vi "Get_LAN_Portnumber.vi"(8 "error in (no error)":errorcluster, 11 ".NET Reference in":refnum<k24>) -> (0 "error out":errorcluster, 1 "portnum":i32, 3 "Reference out":refnum<k24>)   [LabVIEW 2017]
uses:
  C:/Users/Ssantec_Test/Documents/Instrument_DLL_Sample_Labview_20220902_Ver1.2.2/DLL/x86/InstrumentDLL.dll
  DLL/x86/InstrumentDLL.dll
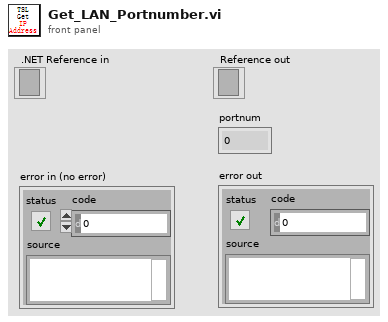
[diagram p1: front panel]
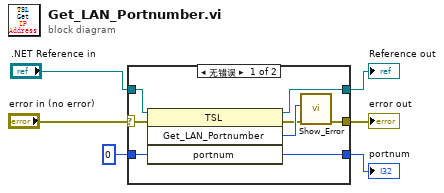
[diagram p0: block diagram]
diagram:
  n1 = case shown="无错误" "error in (no error)" {
    selector: "error in (no error)" -> [w7 w16]
    tunnel: ".NET Reference in" -> [w14 w17]
    tunnel: [w13 w17] -> w5
    tunnel: [w8 w16] -> w4
    tunnel: [w12 w15] -> w3
    tunnel: 0 ("portnum") -> [w11 w15]
    frame No Error {
      n2 = invoke on="调用节点" class="TSL" method="Get_LAN_Portnumber"(reference=w14, error in=w7, "portnum"=w11) -> (reference out=w13:refnum<k24>, error out=w9:errorcluster, "Get_LAN_Portnumber"=w10:i32, "portnum"=w12:i32)  [unwired: 1 in]
      n3 = call "Show_Error.vi"("error in (no error)"=w9, "Error"=w10) -> ("error out"=w8:errorcluster)  [unwired: 9 in]
    }
    frame Error {
    }
  }
  "Reference out" <- w5
  "error out" <- w4
  "portnum" <- w3
